vi "KillTask.vi"(8 "error in (no error)":errorcluster, 11 "Taskname":string) -> (0 "error out":errorcluster)   [LabVIEW 2013, in "main.lvlib"]
uses:
  main.lvlib
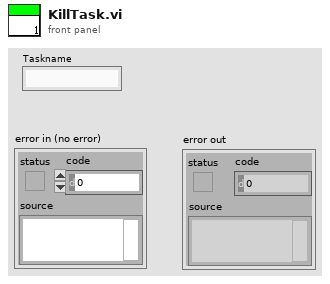
[diagram p1: front panel]
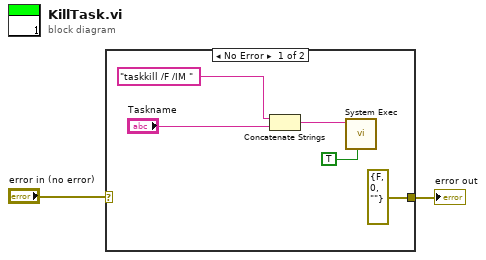
[diagram p0: block diagram]
diagram:
  n1 = case shown="No Error" "error in (no error)" {
    selector: "error in (no error)" -> [_ w8]
    tunnel: [errorcluster {"status"=FALSE, "code"=0, "source"=""} ("error IO") w8] -> w1
    frame No Error {
      n2 = Concatenate Strings("taskkill /F /IM " ("command line"), "Taskname") -> (w5:string)
      n3 = call <vilib>:"System Exec.vi"("run minimized? (F)"=TRUE, "command line"=w5) -> ()  [unwired: 6 in, 4 out]
    }
    frame Error {
    }
  }
  "error out" <- w1
